vi "centroide.vi"(0 "Array 2":u32[][](array[numeric])) -> (1 "cx":u16, 2 "cy":u16)   [LabVIEW 2021]
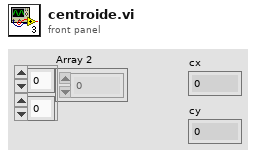
[diagram p1: front panel]
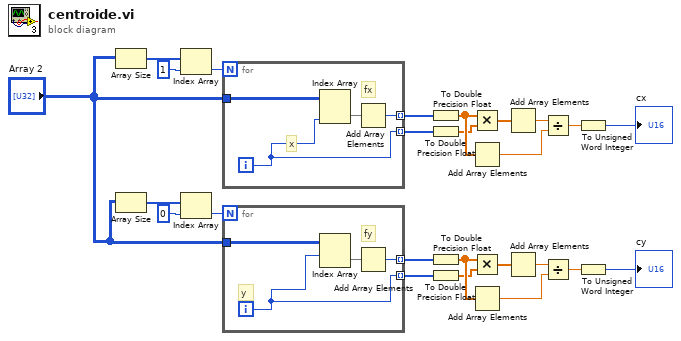
[diagram p0: block diagram]
diagram:
  n1 = Array Size(array="Array 2") -> (size(s)=w15:i32[])
  n2 = Array Size(array="Array 2") -> (size(s)=w3:i32[])
  n3 = Index Array(array=w15, index=1) -> (element=w17:i32)
  n4 = Index Array(array=w3, index=0) -> (element=w5:i32)
  n5 = for {
    N: w17 -> [_]
    tunnel: "Array 2" -> [w29]
    tunnel: [w27] -> w22 mode=indexing
    tunnel: [w26] -> w20 mode=indexing
    i -> [w26]
    # "x"
    # "fx"
    n6 = Index Array(array=w29, index (col)=w26) -> (element=w28:u32[])  [unwired: 1 in]
    n7 = Add Array Elements(numeric array=w28) -> (sum=w27:u32)
  }
  n8 = for {
    N: w5 -> [_]
    tunnel: "Array 2" -> [w33]
    tunnel: [w31] -> w10 mode=indexing
    tunnel: [w30] -> w8 mode=indexing
    i -> [w30]
    # "y"
    # "fy"
    n9 = Index Array(array=w33, index (row)=w30) -> (element=w32:u32[])  [unwired: 1 in]
    n10 = Add Array Elements(numeric array=w32) -> (sum=w31:u32)
  }
  n11 = To Double Precision Float(number=w22) -> (double precision float=w25:dbl[])
  n12 = To Double Precision Float(number=w20) -> (double precision float=w21:dbl[])
  n13 = To Double Precision Float(number=w10) -> (double precision float=w13:dbl[])
  n14 = To Double Precision Float(number=w8) -> (double precision float=w9:dbl[])
  n15 = Multiply(x=w25, y=w21) -> (x*y=w18:dbl[])
  n16 = Add Array Elements(numeric array=w25) -> (sum=w23:dbl)
  n17 = Multiply(x=w13, y=w9) -> (x*y=w6:dbl[])
  n18 = Add Array Elements(numeric array=w13) -> (sum=w11:dbl)
  n19 = Add Array Elements(numeric array=w18) -> (sum=w24:dbl)
  n20 = Add Array Elements(numeric array=w6) -> (sum=w12:dbl)
  n21 = Divide(x=w24, y=w23) -> (x/y=w19:dbl)
  n22 = Divide(x=w12, y=w11) -> (x/y=w7:dbl)
  n23 = To Unsigned Word Integer(number=w19) -> (unsigned 16bit integer=→"cx":u16)
  n24 = To Unsigned Word Integer(number=w7) -> (unsigned 16bit integer=→"cy":u16)
